vi "Watlow Modbus.vi"(6 "Watlow Present?":bool, 7 "Modbus Mode":T2, 8 "Error IN":errorcluster, 10 "Data Write":sgl format="%#_13g", 11 "Variable":T1) -> (0 "Error OUT":errorcluster, 3 "Data Read":sgl)   [LabVIEW 2019]
uses:
  Modbus Mode.ctl
  Modbus Variable.ctl
  NI Modbus.llb/MB Modbus Command.ctl
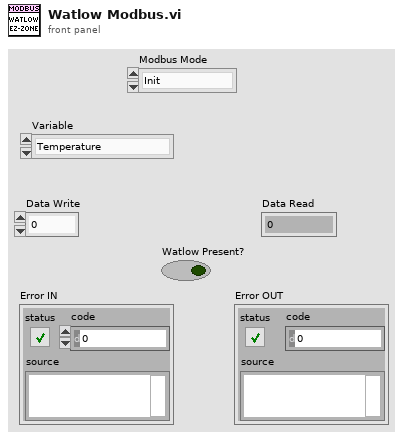
[diagram p1: front panel]
types:
  T1 = typedef "Modbus Variable.ctl" = enum16{"Temperature", "Setpoint"}
  T2 = typedef "Modbus Mode.ctl" = enum16{"Init", "Tank 1 Write", "Tank 2 Write", "Tank 1 Read", "Tank 2 Read"}
  T3 = cluster{"Mode":enum16{"RTU", "ASCII"}, "Slave Address":u8}
  T4 = typedef "MB Modbus Command.ctl" = cluster{"Function Code":u8, "Starting Address":u16, "Quantity":u16, "Data":u16[], "Discrete":bool[]}
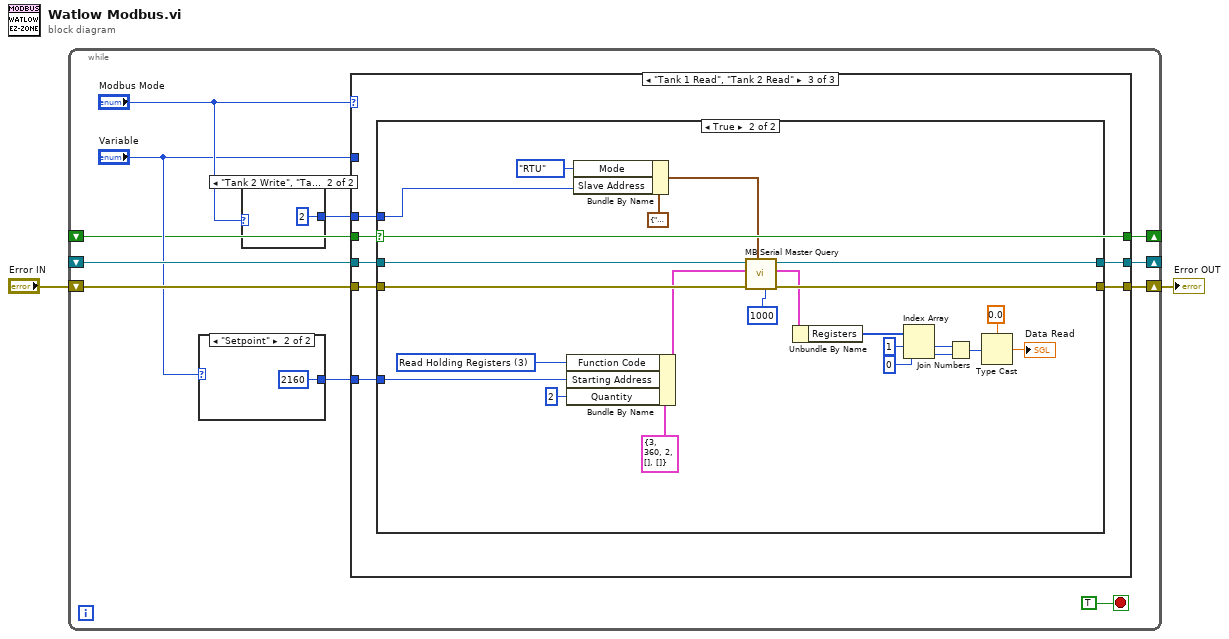
[diagram p0: block diagram]
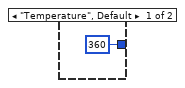
[diagram p2: hidden frame]
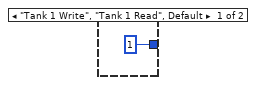
[diagram p3: hidden frame]
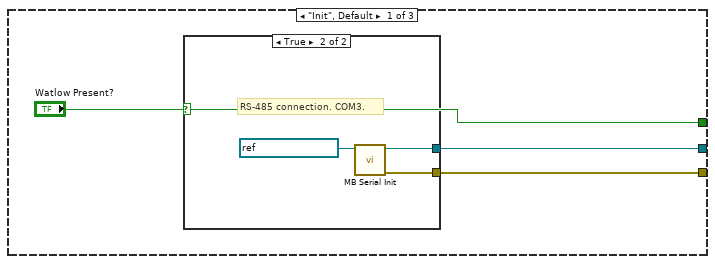
[diagram p4: hidden frame]
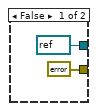
[diagram p5: hidden frame]
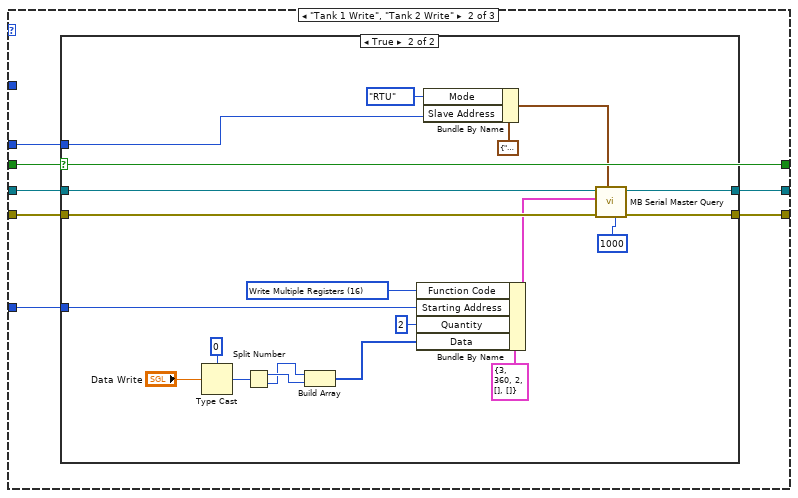
[diagram p6: hidden frame]
diagram:
  n1 = while {
    shift-right: [w12] -> _
    shift-left: _ -> [w10]
    shift-right: [w11] -> w1
    shift-left: "Error IN" -> [w9]
    shift-right: [w4] -> _
    shift-left: _ -> [w3]
    stop <- TRUE stop-if-true
    n2 = case shown="\"Setpoint\"" "Variable" {
      tunnel: [u16 360 ("Starting Address") u16 2160 ("Starting Address")] -> w6
      frame "Temperature", Default {
      }
      frame "Setpoint" {
      }
    }
    n3 = case shown="\"Tank 2 Write\", \"Tank 2 Read\"" "Modbus Mode" {
      tunnel: [u8 1 ("Slave Address") u8 2 ("Slave Address")] -> w7
      frame "Tank 1 Write", "Tank 1 Read", Default {
      }
      frame "Tank 2 Write", "Tank 2 Read" {
      }
    }
    n4 = case shown="\"Tank 1 Read\", \"Tank 2 Read\"" "Modbus Mode" {
      tunnel: "Variable" -> [_ _ _]
      tunnel: [w20 w31 w60] -> w12
      tunnel: [w19 w30 w59] -> w11
      tunnel: w10 -> [_ w32 w61]
      tunnel: w9 -> [_ w29 w58]
      tunnel: w7 -> [_ w28 w57]
      tunnel: w6 -> [_ w27 w56]
      tunnel: ["Watlow Present?" w26 w55] -> w4
      tunnel: w3 -> [_ w26 w55]
      frame "Init", Default {
        n5 = case shown="True" "Watlow Present?" {
          tunnel: [refnum<visa-resource-name> refnum ("VISA resource name out") w24] -> w20
          tunnel: [errorcluster {"status"=FALSE, "code"=0, "source"=""} ("error out") w23] -> w19
          frame False {
          }
          frame True {
            # "RS-485 connection. COM3."
            n6 = call "MB Serial Init.vi"("VISA resource name"=refnum<visa-resource-name> "ASRL3::INSTR") -> ("error out"=w23:errorcluster, "VISA resource name out"=w24:refnum<visa-resource-name>)  [unwired: 6 in, 3 out]
          }
        }
      }
      frame "Tank 1 Write", "Tank 2 Write" {
        n7 = case shown="True" w26 {
          tunnel: w32 -> [w34 w54]
          tunnel: [w34 w53] -> w31
          tunnel: [w33 w52] -> w30
          tunnel: w29 -> [w33 w51]
          tunnel: w28 -> [_ w38]
          tunnel: w27 -> [_ w37]
          frame False {
          }
          frame True {
            w48 = u8 16 items=["Read Coils"=1, "Read Discrete Inputs"=2, "Read Holding Registers"=3, "Read Input Registers"=4, "Write Single Coil"=5, "Write Single Register"=6, "Read Exception Status"=7, "Write Multiple Coils"=15, "Write Multiple Registers"=16] ("Function Code")
            n8 = Type Cast(type=u32 0, x="Data Write") -> (*(type *) &x=w44:u32)
            n9 = Split Number(x=w44) -> (hi(x)=w36:u16, lo(x)=w35:u16)
            n10 = Build Array(w35, w36) -> (w43:u16[])
            n11 = Bundle By Name(cluster=T4 {"Function Code"=3, "Starting Address"=360, "Quantity"=2, "Data"=[], "Discrete"=[]} ("MODBUS Command"), "Function Code"=w48, "Starting Address"=w37, "Quantity"=u16 2, "Data"=w43) -> (w49:T4)
            n12 = Bundle By Name(cluster=T3 {"Mode"=enum."RTU", "Slave Address"=1} ("Serial Parameters"), "Mode"=enum16{"RTU", "ASCII"}."RTU", "Slave Address"=w38) -> (w40:T3)
            n13 = call "MB Serial Master Query.vi"("Timeout"=u32 1000, "Serial Parameters"=w40, "error in (no error)"=w51, "Modbus Command"=w49, "VISA resource name"=w54) -> ("error out"=w52:errorcluster, "VISA resource name out"=w53:refnum<visa-resource-name>)  [unwired: 2 in, 3 out]
          }
        }
      }
      frame "Tank 1 Read", "Tank 2 Read" {
        n14 = case shown="True" w55 {
          tunnel: w61 -> [w63 w86]
          tunnel: [w63 w85] -> w60
          tunnel: [w62 w84] -> w59
          tunnel: w58 -> [w62 w83]
          tunnel: w57 -> [_ w74]
          tunnel: w56 -> [_ w73]
          frame False {
          }
          frame True {
            w80 = u8 3 items=["Read Coils"=1, "Read Discrete Inputs"=2, "Read Holding Registers"=3, "Read Input Registers"=4, "Write Single Coil"=5, "Write Single Register"=6, "Read Exception Status"=7, "Write Multiple Coils"=15, "Write Multiple Registers"=16] ("Function Code")
            n15 = Bundle By Name(cluster=T4 {"Function Code"=3, "Starting Address"=360, "Quantity"=2, "Data"=[], "Discrete"=[]} ("MODBUS Command"), "Function Code"=w80, "Starting Address"=w73, "Quantity"=u16 2) -> (w81:T4)
            n16 = Bundle By Name(cluster=T3 {"Mode"=enum."RTU", "Slave Address"=1} ("Serial Parameters"), "Mode"=enum16{"RTU", "ASCII"}."RTU", "Slave Address"=w74) -> (w76:T3)
            n17 = call "MB Serial Master Query.vi"("Timeout"=u32 1000, "Serial Parameters"=w76, "error in (no error)"=w83, "Modbus Command"=w81, "VISA resource name"=w86) -> ("error out"=w84:errorcluster, "Registers"=w72:cluster{"Registers":u16[], "Discrete":bool[]}, "VISA resource name out"=w85:refnum<visa-resource-name>)  [unwired: 2 in, 2 out]
            n18 = Unbundle By Name(w72) -> ("Registers"=w64:u16[])
            n19 = Index Array(array=w64, index #1=1 ("index"), index #2=0 ("index")) -> (element #1=w65:u16, element #2=w66:u16)
            n20 = Join Numbers(hi=w65, lo=w66) -> ((hi.lo)=w69:u32)
            n21 = Type Cast(type=sgl 0.0 ("single precision float"), x=w69) -> (*(type *) &x=→"Data Read":sgl)
          }
        }
      }
    }
  }
  "Error OUT" <- w1
